vi "Extract Tip Features from Image File.vi"(8 "error in (no error)":errorcluster, 11 "Image Path":path) -> (0 "error out":errorcluster, 3 "Features":dbl[](array[numeric]))   [LabVIEW 2013]
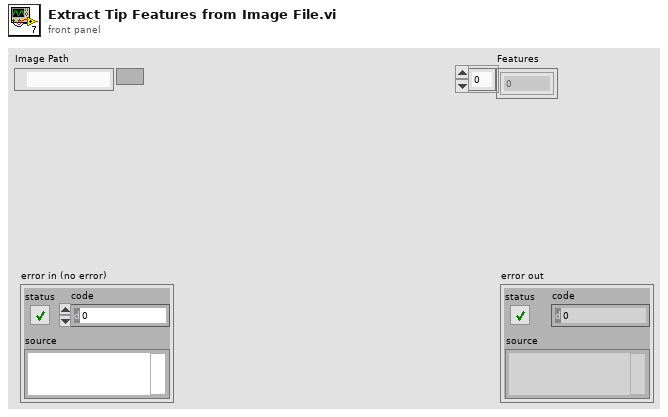
[diagram p1: front panel]
types:
  T1 = typedef "Image Type" = u32
  T2 = typedef "IMAQ Image.ctl" = refnum<image>
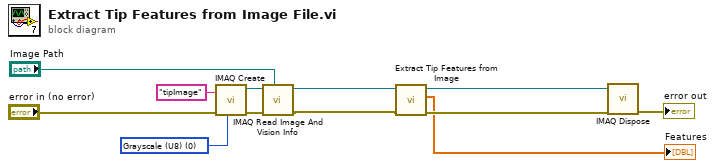
[diagram p0: block diagram]
diagram:
  w9 = T1 0 items=["Grayscale (U8)", "Grayscale (I16)", "Grayscale (SGL)", "Complex (CSG)", "RGB (U32)", "HSL (U32)", "RGB (U64)", "Grayscale (U16)"] ("Image Type")
  n1 = call "IMAQ Create"("Image Name"="tipImage", "Image Type"=w9, "error in (no error)"="error in (no error)") -> ("New Image"=w11:T2, "error out"=w10:errorcluster)  [unwired: 2 in]
  n2 = call "IMAQ Read Image And Vision Info"("File Path"="Image Path", "error in (no error)"=w10, "Image"=w11) -> ("error out"=w4:errorcluster, "Image Out"=w5:T2)  [unwired: 6 in, 1 out]
  n3 = call "Extract Tip Features from Image.vi"("error in (no error)"=w4, "Image In"=w5) -> ("error out"=w2:errorcluster, "Features"=→"Features":dbl[], "Image Out"=w3:T2)  [unwired: 7 in]
  n4 = call "IMAQ Dispose"("Image"=w3, "error in (no error)"=w2) -> ("error out"=→"error out":errorcluster)  [unwired: 4 in]
